vi "MTM2_putSample_axialForce.vi"(8 "error in (no error)":errorcluster, 11 "axialForce_Ctl":T1) -> (0 "error out":errorcluster, 2 "function return":i32, 3 "axialForce_Ctl out":T1)   [LabVIEW 2018, in "SALLV_MTM2.lvlib"]
doc: "int MTM2_shm_putSample_axialForceLV(MTM2_axialForceLV *axialForce_Ctl );"
uses:
  DataTypes/axialForce.ctl
  SALLV_MTM2.lvlib
  SALLV_MTM2.so
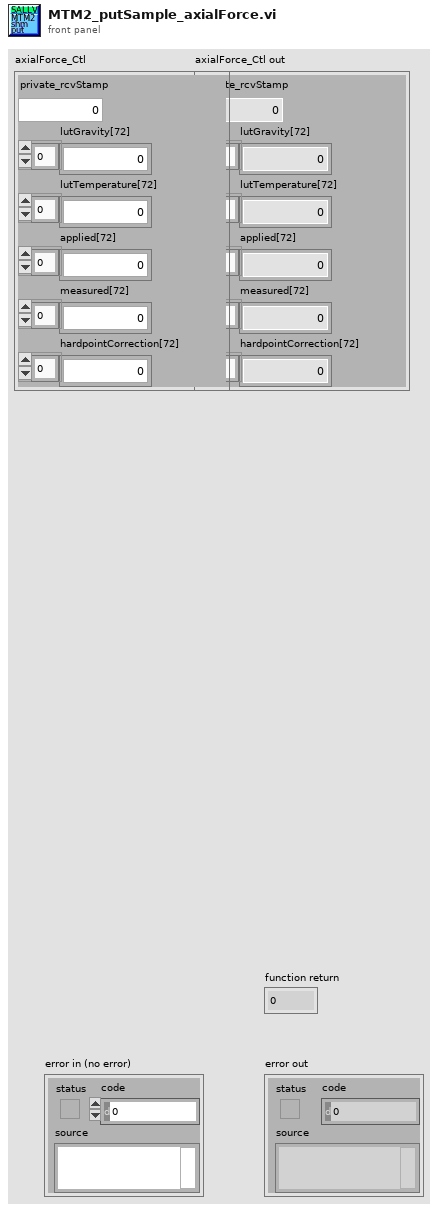
[diagram p1: front panel]
types:
  T1 = typedef "SALLV_MTM2.lvlib/axialForce.ctl" = cluster{"private_rcvStamp":dbl, "lutGravity[72]":dbl[], "lutTemperature[72]":dbl[], "applied[72]":dbl[], "measured[72]":dbl[], "hardpointCorrection[72]":dbl[]}
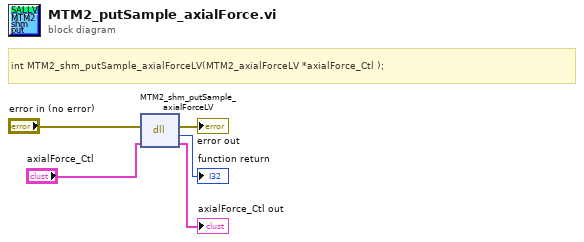
[diagram p0: block diagram]
diagram:
  # "int MTM2_shm_putSample_axialForceLV(MTM2_axialForceLV *axialForce_Ctl );"
  n1 = dll-call lib="home/ttsai/Documents/salTestLabViewApi/SALLV_MTM2/SALLV_MTM2.*" fn="MTM2_shm_putSample_axialForceLV"(error in="error in (no error)", "axialForce_Ctl"="axialForce_Ctl") -> (error out=→"error out":errorcluster, →"function return":i32, "axialForce_Ctl"=→"axialForce_Ctl out":T1)  [unwired: 2 in, 1 out]
